vi "Text To Array1.0.vi"(8 "error in":errorcluster, 11 "file path":path) -> (0 "error out":errorcluster)   [LabVIEW 2013]
doc: "This Function is designed to read in a text file and retunr an array of string with each line of the text file. \n\nFor comments or questions about this code please look at the community example page below.\nhttp://decibel.ni.com/content/docs/DOC-10662"
panel:
  out "array 2":string[](array[string])
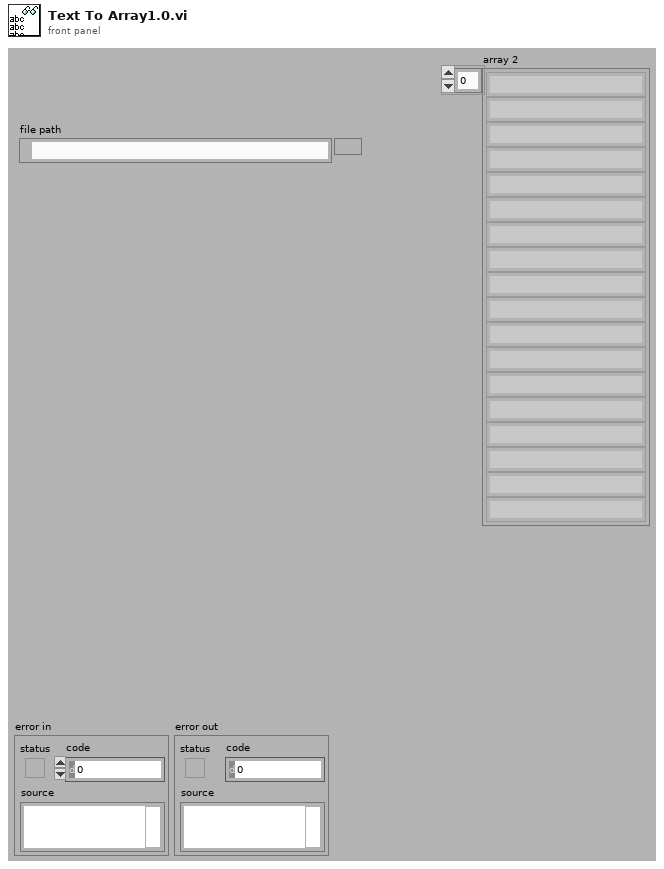
[diagram p1: front panel]
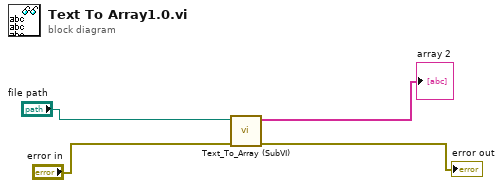
[diagram p0: block diagram]
diagram:
  n1 = call "Text_To_Array (SubVI).vi"("error in (no error)"="error in", "file path"="file path") -> ("error out"=→"error out":errorcluster, "Array"=→"array 2":string[])  [unwired: 8 in]
